vi "processPubDataPublish.vi"(8 "error in (no error)":errorcluster, 11 "MiddlewareSVThisComponent in":refnum<class "MiddlewareSVThisComponent.lvclass">) -> (0 "error out":errorcluster, 3 "MiddlewareSVThisComponent out":refnum<class "MiddlewareSVThisComponent.lvclass">)   [LabVIEW 2015, in "MiddlewareSVThisComponent.lvclass"]
uses:
  MiddlewareSVThisComponent.lvclass
  <vilib>/Utility/error.llb/DialogType.ctl
  ComponentTemplateCore/ComponentModel/ComponentModel/Middleware/Middleware.lvclass
  ComponentTemplateCore/ComponentModel/ComponentModel/MiddlewareProcessEvent/MiddlewareProcessEvent.lvclass
  PubSubDataEvent/PubSubDataEvent.lvclass
  Typedefs/PubDataSV.ctl
  Typedefs/EXATypedefs.lvlib
  Typedefs/CommandValue.ctl
  Typedefs/StateValue.ctl
  Typedefs/RejectedCommand.ctl
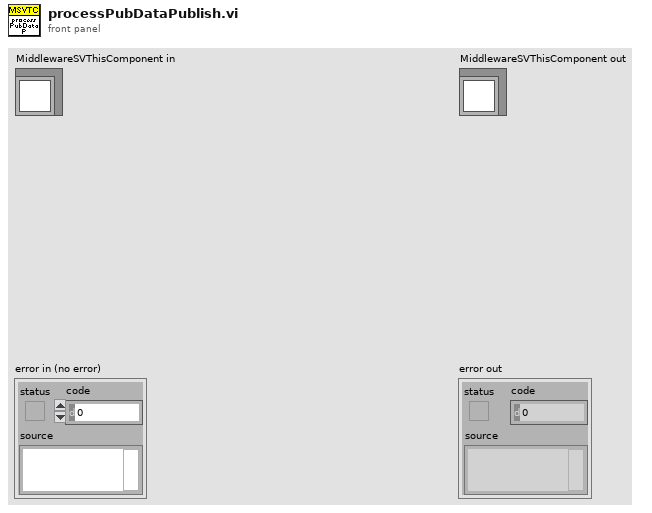
[diagram p1: front panel]
types:
  T1 = typedef "EXATypedefs.lvlib/PubDataEvents.ctl" = cluster{"DetailedState":refnum<user-event>, "ErrorCode":refnum<user-event>, "Heartbeat":refnum<user-event>, "LoopTime_ms":refnum<user-event>, "LoopTimeOutOfRange":refnum<user-event>, "RejectedCommand":refnum<user-event>, "SummaryState":refnum<user-event>, "Timestamp":refnum<user-event>}
  T2 = typedef "MiddlewareProcessEvents.ctl" = cluster{"disconnect":refnum<user-event>, "error":refnum<user-event>}
  T3 = typedef "EXATypedefs.lvlib/PubDataSV.ctl" = enum16{"DetailedState", "ErrorCode", "Heartbeat", "LoopTime_ms", "LoopTimeOutOfRange", "RejectedCommand", "SummaryState", "Timestamp"}
  T4 = typedef "EXATypedefs.lvlib/RejectedCommand.ctl" = cluster{"CommandValue":T5, "StateValue":T6, "Time Stamp":timestamp}
  T5 = typedef "EXATypedefs.lvlib/CommandValue.ctl" = enum16{"ClearError", "Disable", "Enable", "Exit", "GoToStandby", "OnHeartbeat", "OnIncomingMessagingError", "OnInterrupt", "Start"}
  T6 = typedef "EXATypedefs.lvlib/StateValue.ctl" = enum16{"DisabledState", "EnabledState", "FaultState", "OffState", "StandbyState"}
  T7 = typedef "DialogType.ctl" = u16
  T8 = typedef "ComponentStateValues.ctl" = enum16{"Off", "Standby", "Enabled", "Disabled", "Fault"}
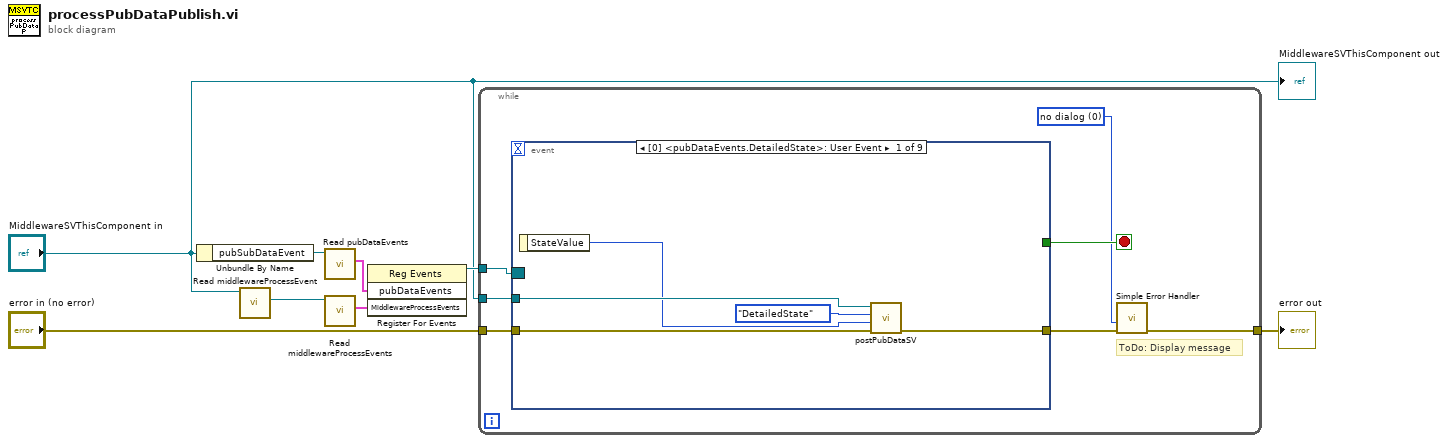
[diagram p0: block diagram]
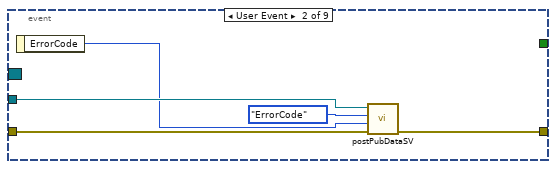
[diagram p2: hidden frame]
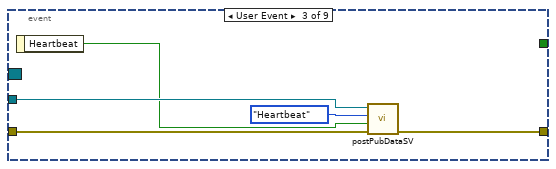
[diagram p3: hidden frame]
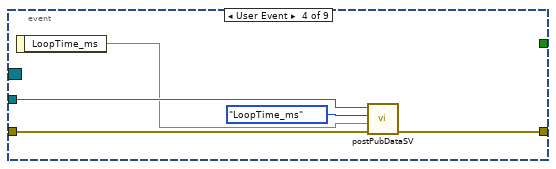
[diagram p4: hidden frame]
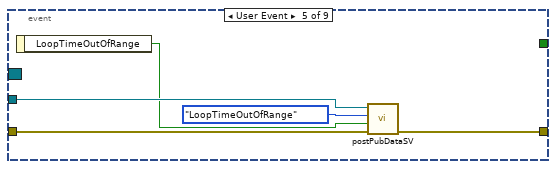
[diagram p5: hidden frame]
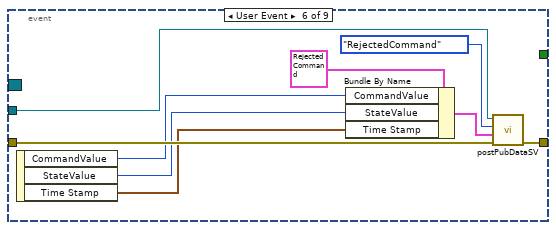
[diagram p6: hidden frame]
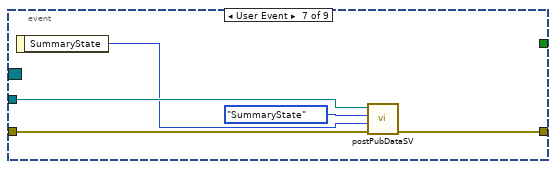
[diagram p7: hidden frame]
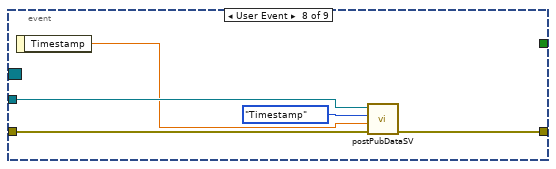
[diagram p8: hidden frame]
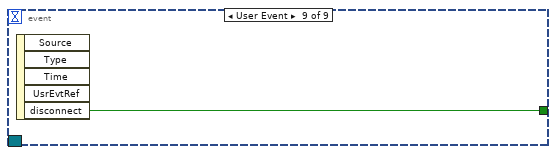
[diagram p9: hidden frame]
diagram:
  n1 = Unbundle By Name("MiddlewareSVThisComponent in") -> ("pubSubDataEvent"=w4:refnum<class "PubSubDataEvent.lvclass">)
  n2 = call "Read middlewareProcessEvent.vi"("Middleware in"="MiddlewareSVThisComponent in") -> ("middlewareProcessEvent"=w6:refnum<class "MiddlewareProcessEvent.lvclass">)  [unwired: 9 in, 1 out]
  n3 = call "Read pubDataEvents.vi"("PubSubDataEvent in"=w4) -> ("pubDataEvents"=w3:T1)  [unwired: 9 in, 1 out]
  n4 = call "Read middlewareProcessEvents.vi"("MiddlewareProcessEvent in"=w6) -> ("MiddlewareProcessEvents"=w5:T2)  [unwired: 9 in, 1 out]
  n5 = register-events(w3, w5) -> (reference out=w8:refnum<event-registration>)  [unwired: 2 in, 1 out]
  n6 = while {
    tunnel: w8 -> [w15]
    tunnel: "error in (no error)" -> [w12]
    tunnel: "MiddlewareSVThisComponent in" -> [w10]
    tunnel: [w9] -> w1
    stop <- w14 stop-if-true
    w13 = T7 0 items=["no dialog", "OK message", "continue or stop message", "OK message + warnings", "continue/stop + warnings"] ("type of dialog (OK msg:1)")
    # "ToDo: Display message"
    n7 = event shown="[0] <pubDataEvents.DetailedState>: User Event" {
      selector: w15 -> [_ _ _ _ _ _ _ _ _]
      dyn-events: _ -> [_ _ _ _ _ _ _ _ _]
      timeout: _ -> [_ _ _ _ _ _ _ _ _]
      tunnel: [_ _ _ _ _ _ _ _ w60] -> w14
      tunnel: w12 -> [w19 w24 w29 w34 w39 w48 w53 w58 _]
      tunnel: [w18 w23 w28 w33 w38 w47 w52 w57 _] -> w11
      tunnel: w10 -> [w20 w25 w30 w35 w40 w49 w54 w59 _]
      event User Event {
        n8 = event-data() -> ("StateValue"=w17:T6)  [unwired: 1 in]
        n9 = call "postPubDataSV.vi"("error in (no error)"=w19, "value"=w17, "pubDataSV"=PubDataSV."DetailedState", "MiddlewareSVThisComponent in"=w20) -> ("error out"=w18:errorcluster)  [unwired: 6 in, 1 out]
      }
      event User Event {
        n10 = event-data() -> ("ErrorCode"=w22:i32)  [unwired: 1 in]
        n11 = call "postPubDataSV.vi"("error in (no error)"=w24, "value"=w22, "pubDataSV"=PubDataSV."ErrorCode", "MiddlewareSVThisComponent in"=w25) -> ("error out"=w23:errorcluster)  [unwired: 6 in, 1 out]
      }
      event User Event {
        n12 = event-data() -> ("Heartbeat"=w27:bool)  [unwired: 1 in]
        n13 = call "postPubDataSV.vi"("error in (no error)"=w29, "value"=w27, "pubDataSV"=PubDataSV."Heartbeat", "MiddlewareSVThisComponent in"=w30) -> ("error out"=w28:errorcluster)  [unwired: 6 in, 1 out]
      }
      event User Event {
        n14 = event-data() -> ("LoopTime_ms"=w32:dbl)  [unwired: 1 in]
        n15 = call "postPubDataSV.vi"("error in (no error)"=w34, "value"=w32, "pubDataSV"=PubDataSV."LoopTime_ms", "MiddlewareSVThisComponent in"=w35) -> ("error out"=w33:errorcluster)  [unwired: 6 in, 1 out]
      }
      event User Event {
        n16 = event-data() -> ("LoopTimeOutOfRange"=w37:bool)  [unwired: 1 in]
        n17 = call "postPubDataSV.vi"("error in (no error)"=w39, "value"=w37, "pubDataSV"=PubDataSV."LoopTimeOutOfRange", "MiddlewareSVThisComponent in"=w40) -> ("error out"=w38:errorcluster)  [unwired: 6 in, 1 out]
      }
      event User Event {
        n18 = event-data() -> ("CommandValue"=w43:T5, "StateValue"=w42:T6, "Time Stamp"=w41:timestamp)  [unwired: 1 in]
        n19 = Bundle By Name(cluster=T4 {"CommandValue"=enum."ClearError", "StateValue"=enum."DisabledState", "Time Stamp"=timestamp(0 s since 1904-01-01)} ("RejectedCommand"), "CommandValue"=w43, "StateValue"=w42, "Time Stamp"=w41) -> (w44:T4)
        n20 = call "postPubDataSV.vi"("error in (no error)"=w48, "value"=w44, "pubDataSV"=PubDataSV."RejectedCommand", "MiddlewareSVThisComponent in"=w49) -> ("error out"=w47:errorcluster)  [unwired: 6 in, 1 out]
      }
      event User Event {
        n21 = event-data() -> ("SummaryState"=w50:T8)  [unwired: 1 in]
        n22 = call "postPubDataSV.vi"("error in (no error)"=w53, "value"=w50, "pubDataSV"=PubDataSV."SummaryState", "MiddlewareSVThisComponent in"=w54) -> ("error out"=w52:errorcluster)  [unwired: 6 in, 1 out]
      }
      event User Event {
        n23 = event-data() -> ("Timestamp"=w55:dbl)  [unwired: 1 in]
        n24 = call "postPubDataSV.vi"("error in (no error)"=w58, "value"=w55, "pubDataSV"=PubDataSV."Timestamp", "MiddlewareSVThisComponent in"=w59) -> ("error out"=w57:errorcluster)  [unwired: 6 in, 1 out]
      }
      event User Event {
        n25 = event-data() -> ("disconnect"=w60:bool)  [unwired: 1 in, 4 out]
      }
    }
    n26 = call <vilib>:"Simple Error Handler.vi"("type of dialog (OK msg:1)"=w13, "error in (no error)"=w11) -> ("error out"=w9:errorcluster)  [unwired: 3 in, 4 out]
  }
  "error out" <- w1
  "MiddlewareSVThisComponent out" <- "MiddlewareSVThisComponent in"
